vi "average data.vi"(6 "state":T2=enum."Process data", 8 "error in (no error)":errorcluster, 10 "data input":dbl[](array[numeric])) -> (0 "error out":errorcluster, 1 "new interval":bool, 2 "averaged data":T3, 3 "total HRT":dbl, 4 "coag model":T1)   [LabVIEW 2015]
uses:
  Sensor buffer command.ctl
  data channels.ctl
  state.ctl
  coag model data.ctl
  ini.ctl
  data ave state.ctl
  data array with time.ctl
  model type.ctl
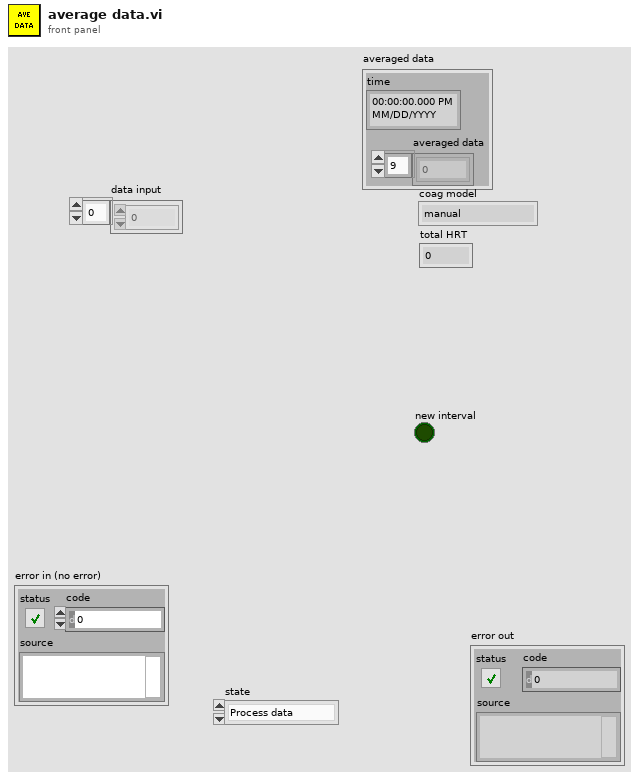
[diagram p1: front panel]
types:
  T1 = typedef "model type.ctl" = enum16{"manual", "ramp", "simple corrector", "linear regression"}
  T2 = typedef "data ave state.ctl" = enum16{"Initialize", "Process data"}
  T3 = typedef "data array with time.ctl" = cluster{"time":timestamp, "averaged data":dbl[]}
  T4 = typedef "Sensor buffer command.ctl" = enum16{"set buffer size", "write", "refill buffer", "read recent", "read all", "clear"}
  T5 = typedef "ini.ctl" = enum16{"write", "read"}
  T6 = typedef "coag model data.ctl" = cluster{"flow rate (L/s)":dbl, "Raw turbidity (NTU)":dbl, "floc sed turbidity (NTU)":dbl}
  T7 = typedef "state.ctl" = enum16{"Initialize", "Process data", "Close"}
  T8 = typedef "data channels.ctl" = enum16{"plant flow [L/s]", "Head Loss [m]", "sludge flow [L/s]", "UV 254", "raw [NTU]", "floc sed [NTU]", "clarified [NTU]", "filtered [NTU]"}
  T9 = typedef "setpoints.ctl" = cluster{"graph data interval (s)":sgl, "sludge flow [L/s]":dbl, "plant flow [L/s]":dbl, "Plant Flow PID ":cluster{"proportional gain (Kc)":dbl, "integral time (Ti, min)":dbl, "derivative time (Td, min)":dbl}, "Sludge PID ":cluster{"proportional gain (Kc)":dbl, "integral time (Ti, min)":dbl, "derivative time (Td, min)":dbl}, "backwash":T10, "Coagulant":T11}
  T10 = typedef "backwash.ctl" = cluster{"Filtered quality target [NTU]":dbl, "min filtration time [s]":dbl, "Ripen time [s]":dbl}
  T11 = typedef "coag.ctl" = cluster{"flocculator volume (L)":dbl, "clarifier volume (L)":dbl, "dose updates per HRT":u16, "target clarified turbidity (NTU)":dbl, "Coagulant mode":T1, "Coag dose [mg/L]":dbl, "pump mL/rev":dbl, "clarifier flow [L/s]":dbl, "min Coag dose [mg/L]":dbl, "max Coag dose [mg/L]":dbl, "Steps":u16, "HRT response delay":u32, "Ku*":dbl}
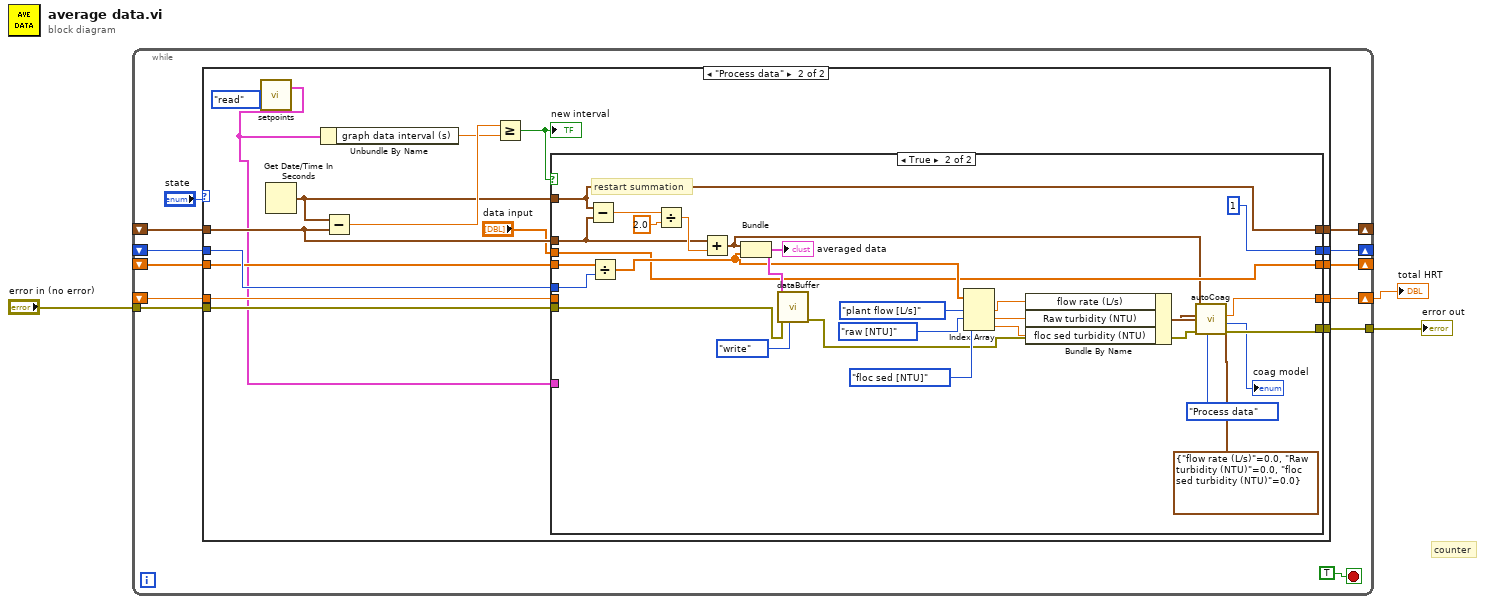
[diagram p0: block diagram]
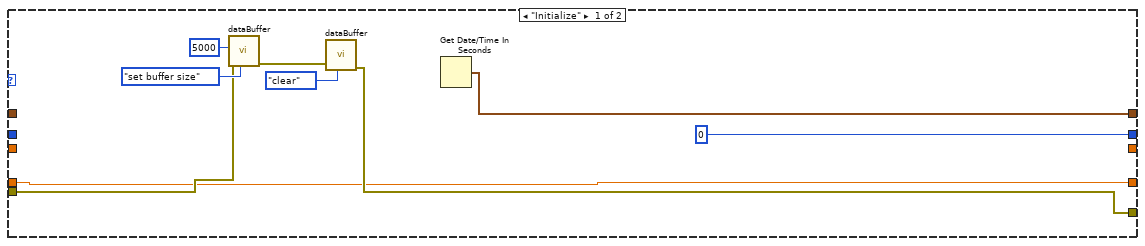
[diagram p2: hidden frame]
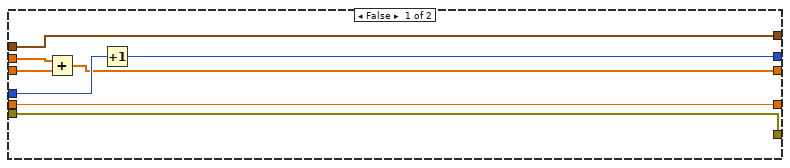
[diagram p3: hidden frame]
diagram:
  # "counter"
  n1 = while {
    shift-right: [w12] -> _
    shift-left: _ -> [w9]
    shift-right: [w14] -> _
    shift-left: _ -> [w13]
    shift-right: [w11] -> _
    shift-left: _ -> [w10]
    tunnel: "error in (no error)" -> [w7]
    tunnel: [w6] -> w2
    shift-right: [w5] -> w1
    shift-left: _ -> [w4]
    stop <- TRUE stop-if-true
    n2 = case shown="\"Process data\"" "state" {
      tunnel: [0 w41] -> w14
      tunnel: w13 -> [_ w40]
      tunnel: [w24 w39] -> w12
      tunnel: [_ w38] -> w11
      tunnel: w10 -> [_ w37]
      tunnel: w9 -> [_ w36]
      tunnel: [w17 w29] -> w6
      tunnel: w7 -> [w18 w30]
      tunnel: [w16 w28] -> w5
      tunnel: w4 -> [w16 w27]
      frame "Initialize" {
        n3 = call "dataBuffer.vi"("command"=Sensor_buffer_command."set buffer size", "error in (no error)"=w18, "max array size"=u16 5000) -> ("error out"=w19:errorcluster)  [unwired: 3 in, 5 out]
        n4 = call "dataBuffer.vi"("command"=Sensor_buffer_command."clear", "error in (no error)"=w19) -> ("error out"=w17:errorcluster)  [unwired: 4 in, 5 out]
        n5 = Get Date/Time In Seconds() -> (seconds since 1Jan1904=w24:timestamp)
      }
      frame "Process data" {
        n6 = call "setpoints.vi"("ini"=ini."read") -> ("Setpoints out"=w25:T9)  [unwired: 9 in, 1 out]
        n7 = Get Date/Time In Seconds() -> (seconds since 1Jan1904=w31:timestamp)
        n8 = Unbundle By Name(w25) -> ("graph data interval (s)"=w34:sgl)
        n9 = Subtract(x=w31, y=w36) -> (x-y=w35:dbl)
        n10 = Greater Or Equal?(x=w35, y=w34) -> (x >= y?=w33:bool)
        "new interval" <- w33
        n11 = case shown="True" w33 {
          tunnel: [w48 1] -> w41
          tunnel: w40 -> [w49 w70]
          tunnel: [w47 w69] -> w39
          tunnel: w31 -> [_ w69]
          tunnel: w36 -> [w47 w71]
          tunnel: [w45 w64] -> w38
          tunnel: w37 -> [w46 w75]
          tunnel: "data input" -> [w44 w64]
          tunnel: w30 -> [w43 w66]
          tunnel: [w43 w57] -> w29
          tunnel: w25 -> [_ _]
          tunnel: [w42 w55] -> w28
          tunnel: w27 -> [w42 _]
          frame False {
            n12 = Add(x=w44, y=w46) -> (x+y=w45:dbl[])
            n13 = Increment(x=w49) -> (x+1=w48:i32)
          }
          frame True {
            # "restart summation"
            n14 = Subtract(x=w69, y=w71) -> (x-y=w73:dbl)
            n15 = Divide(x=w75, y=w70) -> (x/y=w65:dbl[])
            n16 = Divide(x=w73, y=2.0) -> (x/y=w72:dbl)
            n17 = Add(x=w71, y=w72) -> (x+y=w59:timestamp)
            n18 = Bundle(w59, w65) -> (w68:cluster{timestamp, dbl[]})  [unwired: 1 in]
            "averaged data" <- w68
            n19 = call "dataBuffer.vi"("command"=Sensor_buffer_command."write", "error in (no error)"=w66, "averaged data"=w68) -> ("error out"=w58:errorcluster)  [unwired: 3 in, 5 out]
            n20 = Index Array(array=w65, index #1=data_channels."plant flow [L/s]" ("channel"), index #2=data_channels."raw [NTU]" ("channel"), index #3=data_channels."floc sed [NTU]" ("channel")) -> (element #1=w54:dbl, element #2=w51:dbl, element #3=w50:dbl)
            n21 = Bundle By Name(cluster=T6 {"flow rate (L/s)"=0.0, "Raw turbidity (NTU)"=0.0, "floc sed turbidity (NTU)"=0.0} ("data input"), "flow rate (L/s)"=w54, "Raw turbidity (NTU)"=w51, "floc sed turbidity (NTU)"=w50) -> (w52:T6)
            n22 = call "autoCoag.vi"("state"=state."Process data", "current time"=w59, "error in (no error)"=w58, "data input"=w52) -> ("error out"=w57:errorcluster, "coag model"=→"coag model":T1, "total HRT"=w55:dbl)  [unwired: 5 in]
          }
        }
      }
    }
  }
  "error out" <- w2
  "total HRT" <- w1
